vi "Client Read String Until Test.vi"() -> ()   [LabVIEW 2014, in "ESP8266 WiFi Wrapper.lvlib"]
uses:
  ESP8266 WiFi Wrapper.lvlib
panel:
  out "Read String":string
  out "Error Out":errorcluster
  in  "Error In":errorcluster
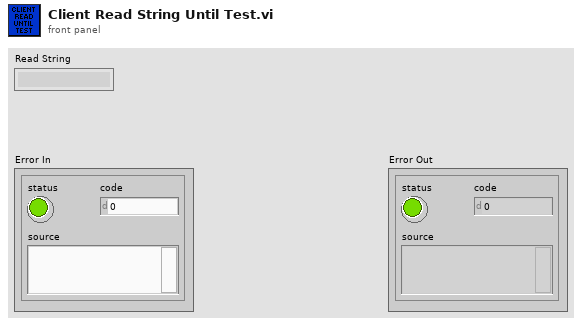
[diagram p1: front panel]
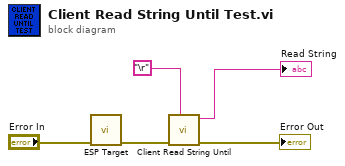
[diagram p0: block diagram]
diagram:
  n1 = call "ESP Target.vi"("Error In"="Error In") -> ("Error Out"=w2:errorcluster)  [unwired: 10 in]
  n2 = call "Client Read String Until.vi"("Terminator char"="\r", "Error In"=w2) -> ("Error Out"=→"Error Out":errorcluster, "Read String"=→"Read String":string)  [unwired: 8 in]
